vi "input.vi"(8 "error in":errorcluster, 10 "input allocation":T1, 11 "GPIC ScaleAndLimit runtime in":refnum<class "GPIC ScaleAndLimit runtime.lvclass">) -> (0 "error out":errorcluster, 2 "input data":T1, 3 "GPIC ScaleAndLimit runtime out":refnum<class "GPIC ScaleAndLimit runtime.lvclass">)   [LabVIEW 2015, in "GPIC ScaleAndLimit runtime.lvclass"]
doc: "Provides an interface for reading data from a module at runtime. While this interface performs no operations, a child should provide an override which may read from any open sessions, references, or interfaces."
uses:
  GPIC ScaleAndLimit runtime.lvclass
  <vilib>/NI/Tag Bus/table/data table.ctl
  GPIC ScaleAndLimit runtime.lvclass/GPIC ScaleAndLimit runtime.ctl
  <vilib>/NI/Tag Bus/table/data table.lvlib
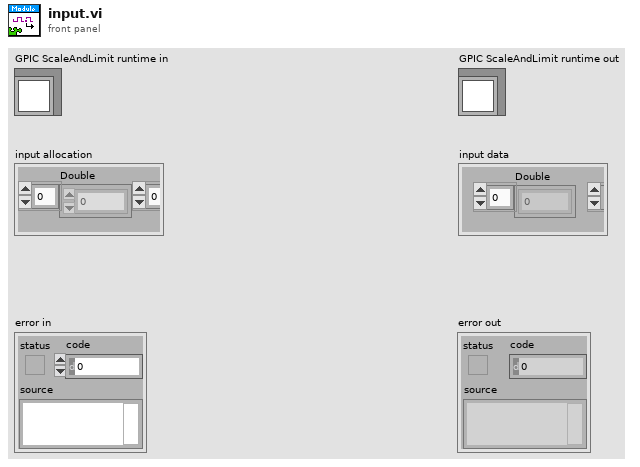
[diagram p1: front panel]
types:
  T1 = typedef "tag bus.lvlib/data table.lvlib/data table.ctl" = cluster{"Double":dbl[], "Single":sgl[], "I64":i64[], "I32":i32[], "I16":i16[], "I8":i8[], "U64":u64[], "U32":u32[], "U16":u16[], "U8":u8[], "Boolean":bool[], "String":string[], "Array of Double":cluster{"DBL Array":dbl[]}[], "Array of Single":cluster{"SGL Array":sgl[]}[], "Array of I64":cluster{"I64 Array":i64[]}[], "Array of I32":cluster{"I32 Array":i32[]}[], "Array of I16":cluster{"I16 Array":i16[]}[], "Array of I8":cluster{"I8 Array":i8[]}[], "Array of U64":cluster{"U64 Array":u64[]}[], "Array of U32":cluster{"U32 Array":u32[]}[], "Array of U16":cluster{"U16 Array":u16[]}[], "Array of U8":cluster{"U8 Array":u8[]}[], "Array of Boolean":cluster{"Boolean Array":bool[]}[], "Array of String":cluster{"String Array":string[]}[]}
  T2 = typedef "GPIC ScaleAndLimit configuration.lvclass/input data indices.ctl" = cluster{"Single.RMC/Simultaneous/AI0":i32, "Single.RMC/Simultaneous/AI1":i32, "Single.RMC/Simultaneous/AI2":i32, "Single.RMC/Simultaneous/AI3":i32, "Single.RMC/Simultaneous/AI4":i32, "Single.RMC/Simultaneous/AI5":i32, "Single.RMC/Simultaneous/AI6":i32, "Single.RMC/Simultaneous/AI7":i32, "Single.RMC/Simultaneous/AI8":i32, "Single.RMC/Simultaneous/AI9":i32, "Single.RMC/Simultaneous/AI10":i32, "Single.RMC/Simultaneous/AI11":i32, "Single.RMC/Simultaneous/AI12":i32, "Single.RMC/Simultaneous/AI13":i32, "Single.RMC/Simultaneous/AI14":i32, "Single.RMC/Simultaneous/AI15":i32, "Boolean.AILimits":i32, "U16.AILimitHigh":i32, "U16.AILimitLow":i32}
  T3 = typedef "ScaleAndLimitInterface.lvlib/FPGAInterface.ctl" = refnum<k20>
  T4 = typedef "GPIC ScaleAndLimit runtime.lvclass/input user data.ctl" = cluster{"RMC/Simultaneous/AI0":sgl, "RMC/Simultaneous/AI1":sgl, "RMC/Simultaneous/AI2":sgl, "RMC/Simultaneous/AI3":sgl, "RMC/Simultaneous/AI4":sgl, "RMC/Simultaneous/AI5":sgl, "RMC/Simultaneous/AI6":sgl, "RMC/Simultaneous/AI7":sgl, "RMC/Simultaneous/AI8":sgl, "RMC/Simultaneous/AI9":sgl, "RMC/Simultaneous/AI10":sgl, "RMC/Simultaneous/AI11":sgl, "RMC/Simultaneous/AI12":sgl, "RMC/Simultaneous/AI13":sgl, "RMC/Simultaneous/AI14":sgl, "RMC/Simultaneous/AI15":sgl, "AILimits":bool, "AILimitHigh":u16, "AILimitLow":u16}
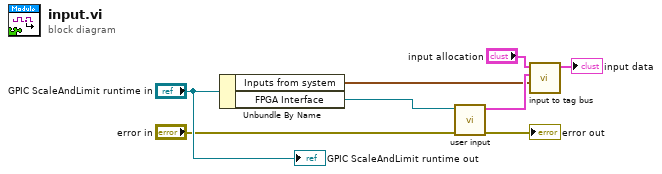
[diagram p0: block diagram]
diagram:
  n1 = Unbundle By Name("GPIC ScaleAndLimit runtime in") -> ("Inputs from system"=w2:T2, "FPGA Interface"=w1:T3)
  n2 = call "user input.vi"("error in"="error in", "FPGA Interface"=w1) -> ("error out"=→"error out":errorcluster, "Inputs from system"=w3:T4)  [unwired: 8 in]
  n3 = call "input to tag bus.vi"("indices"=w2, "data cluster"=w3, "tag bus in"="input allocation") -> ("tag bus out"=→"input data":T1)  [unwired: 8 in]
  "GPIC ScaleAndLimit runtime out" <- "GPIC ScaleAndLimit runtime in"
